vi "Configure Auto Trigger.vi"(6 "Auto Trigger Interval (0.4 s)":dbl=0.4 min=0.008 max=7.0, 7 "Trigger Hold Sensitivity (1: 0.1%)":u16(ring)=1 items=["0.01%", "0.1%", "1%", "10%"], 8 "error in (no error)":errorcluster, 10 "Enable Auto Trigger Hold (Disable)":bool, 11 "VISA resource name":refnum<visa-resource-name>) -> (0 "error out":errorcluster, 3 "VISA resource name out":refnum<visa-resource-name>)   [LabVIEW 2020, in "Library Instrument & Equipement.lvlib" / "Library Multimeter.lvlib" / "RIGOL DM3058.lvlib"]
doc: "Configures the Auto Trigger parameter, include \"Enable Auto Trigger Hold\",\"Trigger Hold Sensitivity\" and \"Auto Trigger Interval\""
uses:
  RIGOL DM3058.lvlib
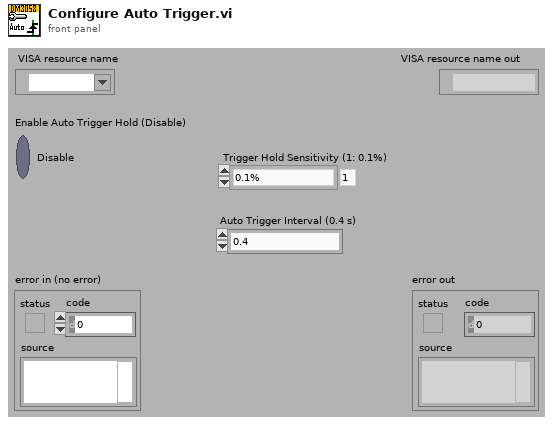
[diagram p1: front panel]
types:
  T1 = cluster{"DM Series Mode":u16, "Measurement Function":u16}
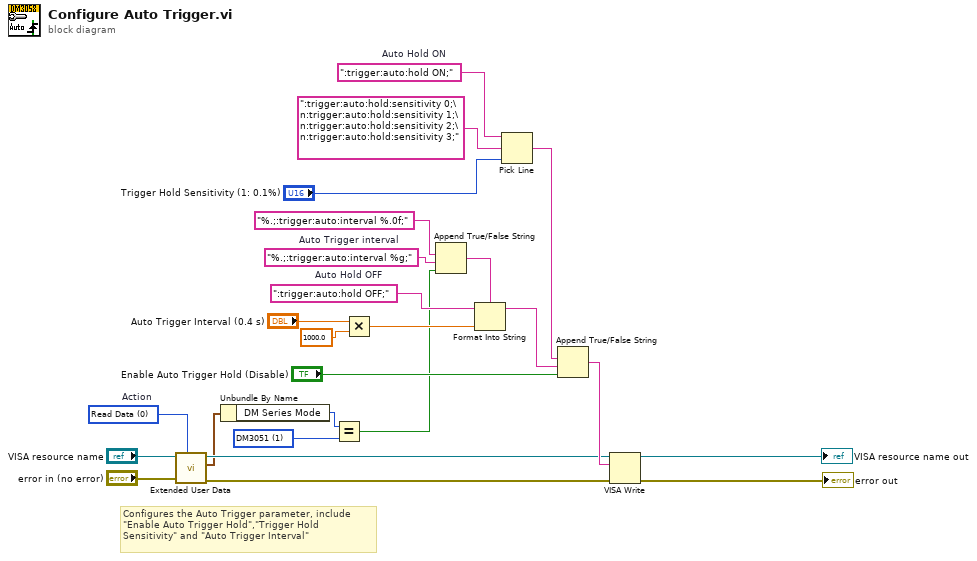
[diagram p0: block diagram]
diagram:
  w2 = u16 1 items=["DM3058", "DM3051", "DM3068", "DM3058E"] ("DM Series Mode")
  w8 = 0 items=["Read Data", "Write Data", "Clear Data", "Clear ALL Data"]  # Action
  w18 = ":trigger:auto:hold OFF;"  # Auto Hold OFF
  w19 = ":trigger:auto:hold ON;"  # Auto Hold ON
  w6 = "%.;:trigger:auto:interval %g;"  # Auto Trigger interval
  # "Configures the Auto Trigger parameter, include \n\"Enable Auto Trigger Hold\",\"Trigger Hold \nSensitivity\" and \"Auto Trigger Interval\""
  n1 = call "Extended User Data.vi"("Action (1: Write Data)"=w8, "Error In (no error)"="error in (no error)", "VISA resource name in"="VISA resource name") -> ("Error Out"=w9:errorcluster, "User Data Out"=w1:T1, "VISA resource name out"=w10:refnum<visa-resource-name>)  [unwired: 1 in, 5 out]
  n2 = Unbundle By Name(w1) -> ("DM Series Mode"=w7:u16)
  n3 = Equal?(x=w7, y=w2) -> (x = y?=w4:bool)
  n4 = Multiply(x="Auto Trigger Interval (0.4 s)", y=1000.0) -> (x*y=w24:dbl)
  n5 = Append True/False String(1:w4, 2:w6, 3:"%.;:trigger:auto:interval %.0f;" ("true string")) -> (0:w5:string)  [unwired: 1 out]
  n6 = Format Into String(format string=w5, initial string=w18, w24) -> (resulting string=w16:string)  [unwired: 1 in, 1 out]
  n7 = Pick Line(string ("")=w19, multi-line string=":trigger:auto:hold:sensitivity 0;\n:trigger:auto:hold:sensitivity 1;\n:trigger:auto:hold:sensitivity 2;\n:trigger:auto:hold:sensitivity 3;", line index="Trigger Hold Sensitivity (1: 0.1%)") -> (output string=w17:string)
  n8 = Append True/False String(1:"Enable Auto Trigger Hold (Disable)", 2:w16, 3:w17) -> (0:w15:string)  [unwired: 1 out]
  n9 = VISA Write(VISA resource name=w10, write buffer=w15, error in (no error)=w9) -> (VISA resource name out=→"VISA resource name out":refnum<visa-resource-name>, error out=→"error out":errorcluster)  [unwired: 1 out]
